vi "Build JSON Path.vi"(10 "Child element":string, 11 "Base $Path":string) -> (3 "$Path out":string)   [LabVIEW 2019, in "JSON-Schema.lvlib"]
uses:
  JSON-Schema.lvlib
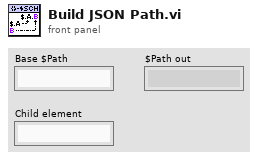
[diagram p1: front panel]
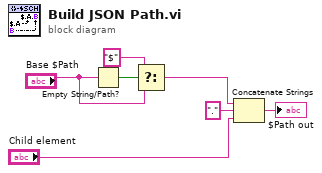
[diagram p0: block diagram]
diagram:
  n1 = Empty String/Path?(string/path="Base $Path") -> (empty?=w4:bool)
  n2 = Select(t="$", s=w4, f="Base $Path") -> (s? t:f=w2:string)
  n3 = Concatenate Strings(w2, "." ("string"), "Child element") -> (→"$Path out":string)
